vi "Disconnect Scope.vi"(2 "error in (no error)":errorcluster, 3 "Scope Model":T1=enum."Tek TDS 694C", 4 "Scope Address":refnum<visa-resource-name>) -> (0 "error out":errorcluster)   [LabVIEW 2020]
uses:
  Typedefs/Scope Models.ctl
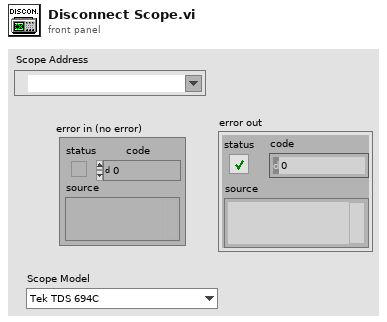
[diagram p1: front panel]
types:
  T1 = typedef "Scope Models.ctl" = enum16{"Tek TDS 684A/B/C", "Tek TDS 694C", "Tek TDS 744/A", "Tek TDS 754A/C/D", "Tek TDS 784A/C/D"}
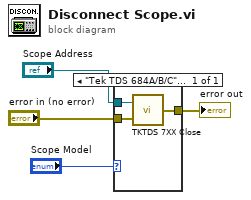
[diagram p0: block diagram]
diagram:
  n1 = case shown="\"Tek TDS 684A/B/C\", Default" "Scope Model" {
    tunnel: "Scope Address" -> [w7]
    tunnel: "error in (no error)" -> [w6]
    tunnel: [w5] -> w1
    frame "Tek TDS 684A/B/C", Default {
      n2 = call <instrlib>:"TKTDS 7XX Close.vi"("error in (no error)"=w6, "VISA session"=w7) -> ("error out"=w5:errorcluster)
    }
  }
  "error out" <- w1
